vi "matlab_TI2_moveToXY.vi"(8 "error in":errorcluster, 10 "yset":dbl, 11 "xset":dbl) -> (0 "error out":errorcluster, 2 "XYZpos":cluster{dbl, dbl, dbl})   [LabVIEW 2018]
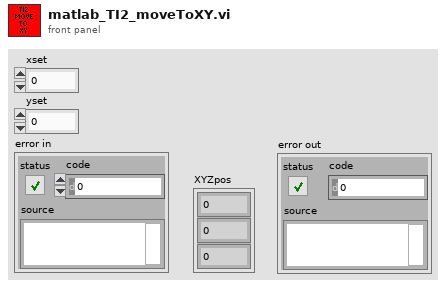
[diagram p1: front panel]
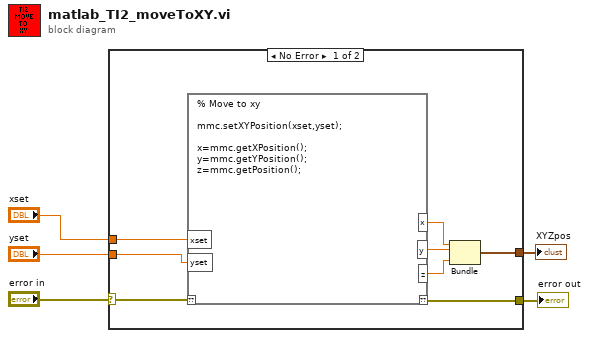
[diagram p0: block diagram]
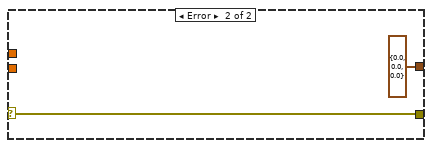
[diagram p2: hidden frame]
diagram:
  n1 = case shown="No Error" "error in" {
    selector: "error in" -> [w13 w15]
    tunnel: [w12 w15] -> w4
    tunnel: "xset" -> [w11 _]
    tunnel: "yset" -> [w10 _]
    tunnel: [w6 cluster{dbl, dbl, dbl} {0.0, 0.0, 0.0}] -> w3
    frame No Error {
      n2 = script code="% Move to xy\n\nmmc.setXYPosition(xset,yset);\n\nx=mmc.getXPosition();\ny=mmc.getYPosition();\nz=mmc.getPosition();"("??"=w13, "xset"=w11, "yset"=w10) -> ("??"=w12:errorcluster, "x"=w8:dbl, "y"=w9:dbl, "z"=w7:dbl)
      n3 = Bundle(w8, w9, w7) -> (w6:cluster{dbl, dbl, dbl})  [unwired: 1 in]
    }
    frame Error {
    }
  }
  "error out" <- w4
  "XYZpos" <- w3
